vi "计算结果-归零试验.vi"(5 "油动机试验路径":path=path "C:/Users/Xiang MU/Desktop/实验文件夹/DR96-16-6203-020/GV1") -> (0 "计算参数 out":T1, 1 "输入参数":T2, 2 "波形图":cluster{dbl, dbl, dbl[][]}(graph))   [LabVIEW 2013]
uses:
  <vilib>/Analysis/3filter.llb/Filter Passband Type.ctl
  <vilib>/Utility/config.llb/Read Key (String).vi
  <vilib>/Analysis/3filter.llb/Butterworth Filter (DBL).vi
  <vilib>/Analysis/NI_AALBase.lvlib
  <vilib>/Utility/config.llb/NI_LVConfig.lvlib
panel:
  in  "计算参数":T1
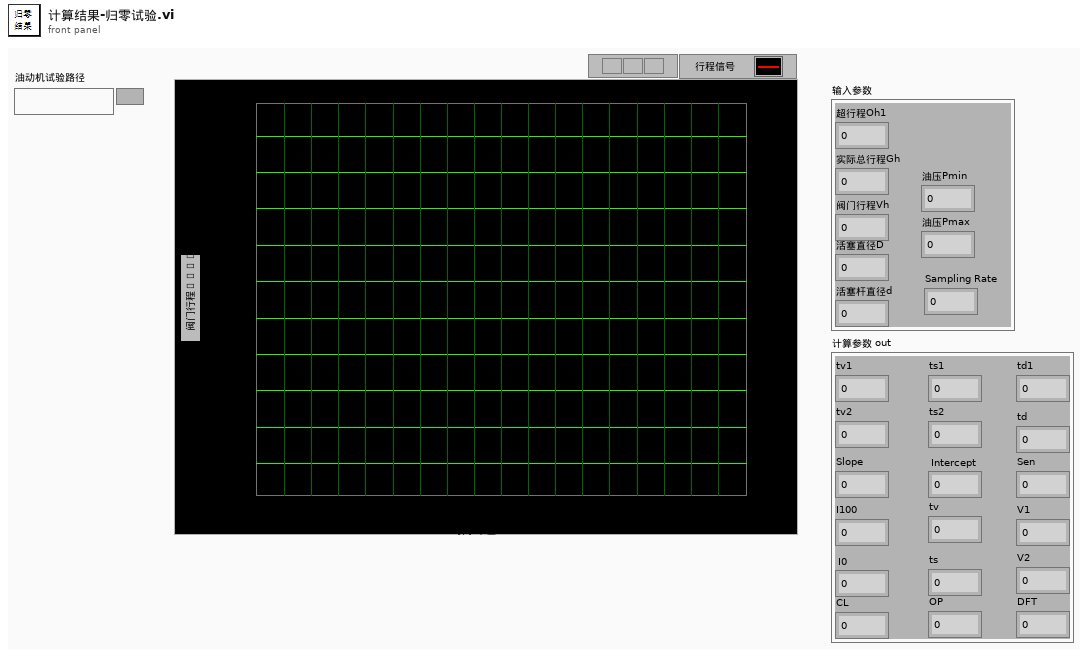
[diagram p1: front panel]
types:
  T1 = cluster{"tv1":dbl, "tv2":dbl, "tv":dbl, "ts1":dbl, "ts2":dbl, "ts":dbl, "td1":dbl, "td":dbl, "Slope":dbl, "Intercept":dbl, "I100":dbl, "I0":dbl, "Sen":dbl, "V1":dbl, "V2":dbl, "CL":dbl, "OP":dbl, "DFT":dbl}
  T2 = cluster{"超行程Oh1":dbl, "实际总行程Gh":dbl, "阀门行程Vh":dbl, "活塞直径D":dbl, "活塞杆直径d":dbl, "油压Pmin":dbl, "油压Pmax":dbl, "Sampling Rate":dbl}
  T3 = typedef "NI_AALBase.lvlib/Filter Passband Type.ctl" = enum32{"Lowpass", "Highpass", "Bandpass", "Bandstop"}
  T4 = typedef "NI_LVConfig.lvlib/Config Data RefNum.ctl" = refnum<k1>
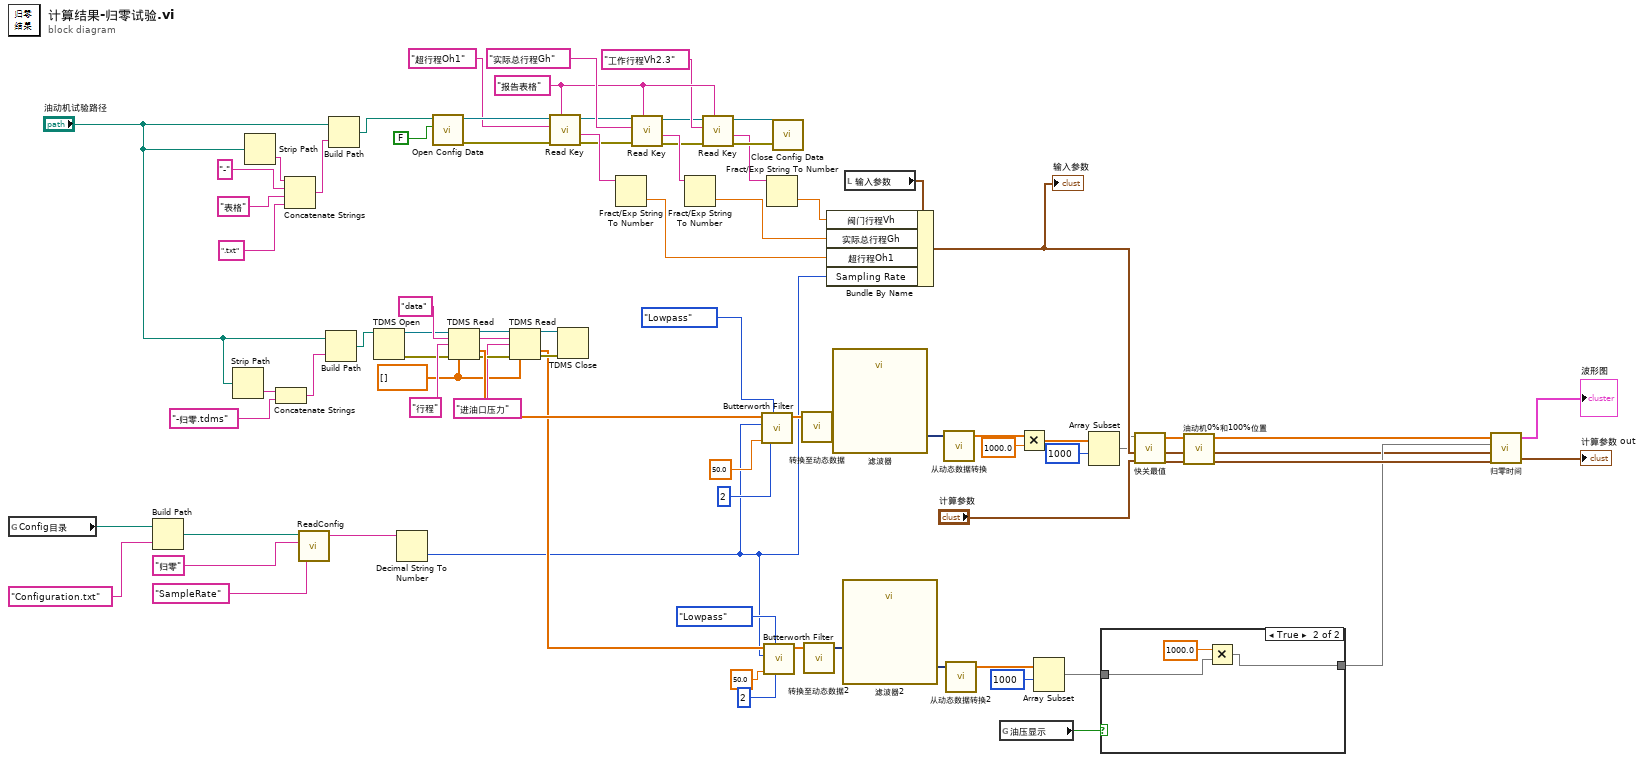
[diagram p0: block diagram]
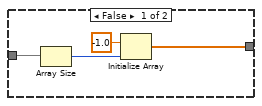
[diagram p2: hidden frame]
diagram:
  w67 = "报告表格" ("key")
  w8 = dbl[] []
  n1 = global read "Config目录.vi" "Config目录"() -> (w24:path)
  n2 = Build Path(base path=w24, name or relative path="Configuration.txt") -> (appended path=w23:path)
  n3 = Strip Path(path="油动机试验路径") -> (name=w41:string)  [unwired: 1 out]
  n4 = Strip Path(path="油动机试验路径") -> (name=w36:string)  [unwired: 1 out]
  n5 = Concatenate Strings(w41, "-归零.tdms") -> (w39:string)
  n6 = Concatenate Strings(w36, "-" ("string"), "表格" ("string"), ".txt") -> (w32:string)
  n7 = call "ReadConfig.vi"("Key"="SampleRate", "Section"="归零", "Path"=w23) -> ("Value"=w28:string)  [unwired: 1 in, 2 out]
  n8 = Build Path(base path="油动机试验路径", name or relative path=w39) -> (appended path=w38:path)
  n9 = Build Path(base path="油动机试验路径", name or relative path=w32) -> (appended path=w31:path)
  n10 = TDMS Open(11:w38) -> (0:w43:errorcluster, 3:w42:refnum<k34>)  [unwired: 6 in]
  n11 = Decimal String To Number(string=w28) -> (number=w3:i32)  [unwired: 2 in, 1 out]
  n12 = call <vilib>:"Open Config Data.vi"("create file if necessary (T)"=FALSE, "configuration file path"=w31) -> ("error out"=w66:errorcluster, "refnum"=w65:T4)  [unwired: 7 in, 1 out]
  n13 = TDMS Read(0:w42, 5:"data" ("组名称输入"), 7:"行程" ("通道名输入"), 11:w43, 12:w8) -> (4:w22:refnum<k34>, 6:w21:string, 10:w50:dbl[], 15:w20:errorcluster)  [unwired: 3 in, 2 out]
  n14 = TDMS Read(0:w22, 5:w21, 7:"进油口压力" ("通道名输入"), 11:w20, 12:w8) -> (4:w17:refnum<k34>, 10:w9:dbl[], 15:w18:errorcluster)  [unwired: 3 in, 3 out]
  n15 = call-poly <vilib>:"Read Key.vi"("section"=w67, "error in (no error)"=w66, "key"="超行程Oh1", "refnum"=w65) -> ("error out"=w61:errorcluster, "value"=w63:string, "refnum out"=w62:T4)  [unwired: 4 in, 1 out]
  n16 = TDMS Close(8:w18, 11:w17) -> ()  [unwired: 2 out]
  n17 = Fract/Exp String To Number(string=w63) -> (number=w74:dbl)  [unwired: 3 in, 1 out]
  n18 = call-poly <vilib>:"Read Key.vi"("section"=w67, "error in (no error)"=w61, "key"="实际总行程Gh", "refnum"=w62) -> ("error out"=w57:errorcluster, "value"=w60:string, "refnum out"=w58:T4)  [unwired: 4 in, 1 out]
  n19 = Fract/Exp String To Number(string=w60) -> (number=w73:dbl)  [unwired: 3 in, 1 out]
  n20 = call-poly <vilib>:"Read Key.vi"("section"=w67, "error in (no error)"=w57, "key"="工作行程Vh2.3", "refnum"=w58) -> ("error out"=w68:errorcluster, "value"=w56:string, "refnum out"=w69:T4)  [unwired: 4 in, 1 out]
  n21 = call-poly <vilib>:"Butterworth Filter.vi"("order"=2, "filter type"=Filter_Passband_Type."Lowpass", "low cutoff freq: fl"=50.0, "sampling freq: fs"=w3, "X"=w50) -> ("Filtered X"=w47:dbl[])  [unwired: 3 in, 1 out]
  n22 = call-poly <vilib>:"Butterworth Filter.vi"("order"=2, "filter type"=Filter_Passband_Type."Lowpass", "low cutoff freq: fl"=50.0, "sampling freq: fs"=w3, "X"=w9) -> ("Filtered X"=w13:dbl[])  [unwired: 3 in, 1 out]
  n23 = Fract/Exp String To Number(string=w56) -> (number=w72:dbl)  [unwired: 3 in, 1 out]
  n24 = call <vilib>:"Close Config Data.vi"("error in (no error)"=w68, "refnum"=w69) -> ()  [unwired: 8 in, 2 out]
  n25 = call "转换至动态数据"("Array"=w47) -> ("Dynamic Data Type"=w48:dynamicdata)  [unwired: 3 in]
  n26 = call "转换至动态数据2"("Array"=w13) -> ("Dynamic Data Type"=w14:dynamicdata)  [unwired: 3 in]
  n27 = call "滤波器"("Signal"=w48) -> ("Filtered Signal"=w49:dynamicdata)  [unwired: 9 in, 1 out]
  n28 = call "滤波器2"("Signal"=w14) -> ("Filtered Signal"=w15:dynamicdata)  [unwired: 9 in, 1 out]
  n29 = local read "输入参数"() -> (w70:T2)
  n30 = Bundle By Name(cluster=w70, "阀门行程Vh"=w72, "实际总行程Gh"=w73, "超行程Oh1"=w74, "Sampling Rate"=w3) -> (w80:T2)
  "输入参数" <- w80
  n31 = call "从动态数据转换"("Dynamic Data Type"=w49) -> ("Array"=w52:dbl[])  [unwired: 3 in]
  n32 = call "从动态数据转换2"("Dynamic Data Type"=w15) -> ("Array"=w6:dbl[])  [unwired: 3 in]
  n33 = global read "油压显示.vi" "油压显示"() -> (w7:bool)
  n34 = Multiply(x=w52, y=1000.0) -> (x*y=w76:dbl[])
  n35 = Array Subset(array=w6, index=1000 ("索引")) -> (w5:dbl[])  [unwired: 1 in]
  n36 = Array Subset(array=w76, index=1000 ("索引")) -> (w79:dbl[])  [unwired: 1 in]
  n37 = case shown="True" w7 {
    tunnel: w5 -> [w87 w89]
    tunnel: [w84 w88] -> w4
    frame False {
      n38 = Array Size(array=w87) -> (size(s)=w86:i32)
      n39 = Initialize Array(-1.0 ("element"), w86) -> (w84:dbl[])
    }
    frame True {
      n40 = Multiply(x=1000.0 ("low cutoff freq: fl"), y=w89) -> (x*y=w88:dbl[])
    }
  }
  n41 = call "快关最值.vi"("计算参数 in"="计算参数", "输入参数 in"=w80, "Array in"=w79) -> ("计算参数 out"=w81:T1, "输入参数 out"=w2:T2, "Array out"=w82:dbl[])  [unwired: 2 in]
  n42 = call "油动机0%和100%位置.vi"("计算参数 in"=w81, "输入参数 in"=w2, "Array in"=w82) -> ("计算参数 out"=w78:T1, "输入参数 out"=w1:T2, "Array out"=w77:dbl[])  [unwired: 2 in]
  n43 = call "归零时间.vi"("计算参数 in"=w78, "输入参数 in"=w1, "进油口压力"=w4, "Array in"=w77) -> ("计算参数 out"=→"计算参数 out":T1, "Waveform Graph"=→"波形图":cluster{dbl, dbl, dbl[][]})  [unwired: 1 in]
